vi "SuperSampleMaster.vi"() -> ()   [LabVIEW 2015]
doc: "A sample master that can be run on the computer or RIO"
panel:
  in  "Show Web":bool
  out "time":string
  out "Status":string
  in  "stop":bool
  # "Instructions:\n1. Run the VI\n2. Verify that you see the correct time."
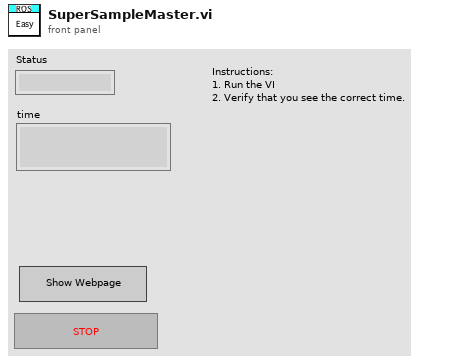
[diagram p1: front panel]
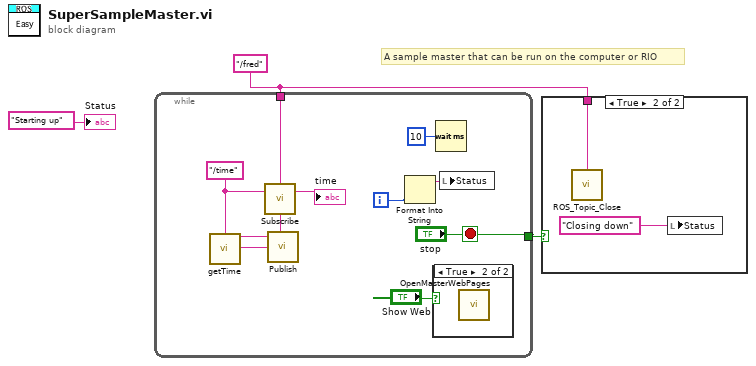
[diagram p0: block diagram]
diagram:
  w1 = "/fred" ("Topic")
  # "A sample master that can be run on the computer or RIO"
  n1 = while {
    tunnel: ["stop"] -> w2
    tunnel: w1 -> [w7]
    i -> [w5]
    stop <- "stop" stop-if-true
    w8 = "/time" ("Topic")
    n2 = call "getTime.vi"() -> ("Current Time"=w9:string)  [unwired: 1 in]
    n3 = call "Subscribe.vi"("Topic"=w8, "node"=w7) -> ("Reply"=→"time":string)  [unwired: 1 in, 1 out]
    n4 = call "Publish.vi"("Topic"=w8, "node"=w7, "String"=w9) -> ()  [unwired: 4 in, 1 out]
    n5 = Format Into String(w5) -> (resulting string=w11:string)  [unwired: 3 in, 1 out]
    n6 = case shown="True" "Show Web" {
      frame False {
      }
      frame True {
        n7 = call "OpenMasterWebPages.vi"() -> ()  [unwired: 4 in]
      }
    }
    n8 = Wait (ms)(milliseconds to wait=u32 10) -> ()  [unwired: 1 out]
    n9 = local write "Status"(w11) -> ()
  }
  n10 = case shown="True" w2 {
    tunnel: w1 -> [_ w13]
    frame False {
    }
    frame True {
      n11 = call "ROS_Topic_Close.vi"("node"=w13) -> ()  [unwired: 3 in, 1 out]
      n12 = local write "Status"("Closing down" ("Status")) -> ()
    }
  }
  "Status" <- "Starting up" ("Status")
